vi "Emballage_BDD_Certificat_S1220009.vi"(0 "CODE BARRE":string, 11 "error in (no error)":errorcluster) -> (4 "Saved Report Path":path=path "C:/Users/ltinguely/Desktop/test model certificat calibration CHIPREG/CHIPREG_Certif_cali__2019-02-14_083035.doc", 15 "error out":errorcluster)   [LabVIEW 2020]
uses:
  Modules/FS/60_FS_Controles/60_FS_SetGet.ctl
  <vilib>/Utility/NIReport.llb/Report Type.ctl
  <vilib>/Utility/NIReport.llb/NI_report.lvclass
  <vilib>/Utility/NIReport.llb/NI_ReportGenerationCore.lvlib
  <vilib>/Utility/NIReport.llb/Word/NI_Word.lvclass
panel:
  out "Temps [s] 2":dbl
  out "Temps [s]":dbl
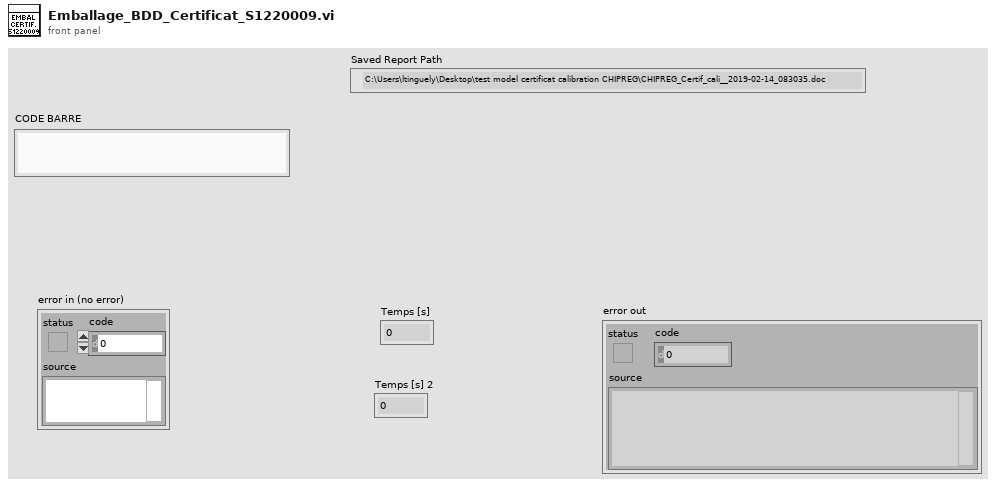
[diagram p1: front panel]
types:
  T1 = typedef "60_FS_SetGet.ctl" = enum16{"set", "get"}
  T2 = enum16{"maximized", "minimized", "normal", "no change"}
  T3 = typedef "NI_ReportGenerationCore.lvlib/Report Type.ctl" = enum16{"HTML", "Word", "Excel"}
  T4 = typedef "60_FS_CLT_Chemins.ctl" = cluster{"Racine_local":path, "Racine_reseau":path, "Racine_Support_Application":path, "Fichier_Journalisation":path, "Connexion_BDD_VSX":path, "Connexion_BDD_PLZ":path}
  T5 = typedef "Emballage_BDD_param_Produit.ctl" = cluster{"No_Valve_FAS":string, "suffixe":string, "designation":string, "indice_produit":string, "code_barre_fixe":string, "affiche_code_barre_client":string, "affiche_no_client":string, "Nb_vlve_par_carton":u16, "melange_des_lots_possible":string, "id_article":string, "Indice_Rev":string, "Famille":string, "date":string, "code_barre_fixe_Fin":string, "Longeur_No_Serie":string}
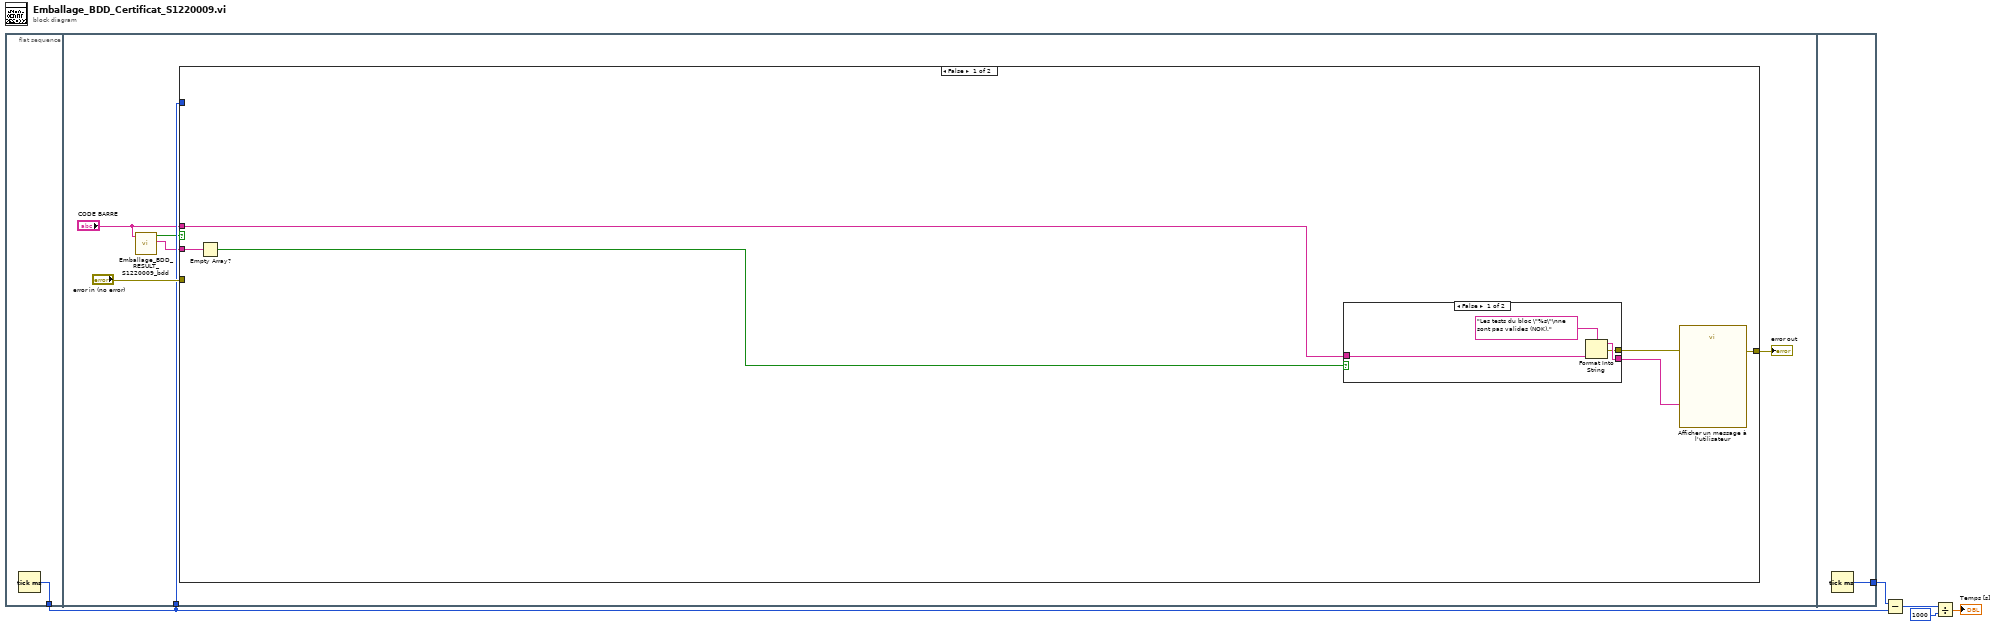
[diagram p0: block diagram]
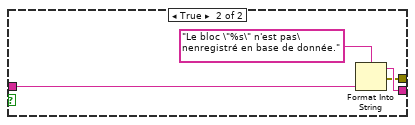
[diagram p2: hidden frame]
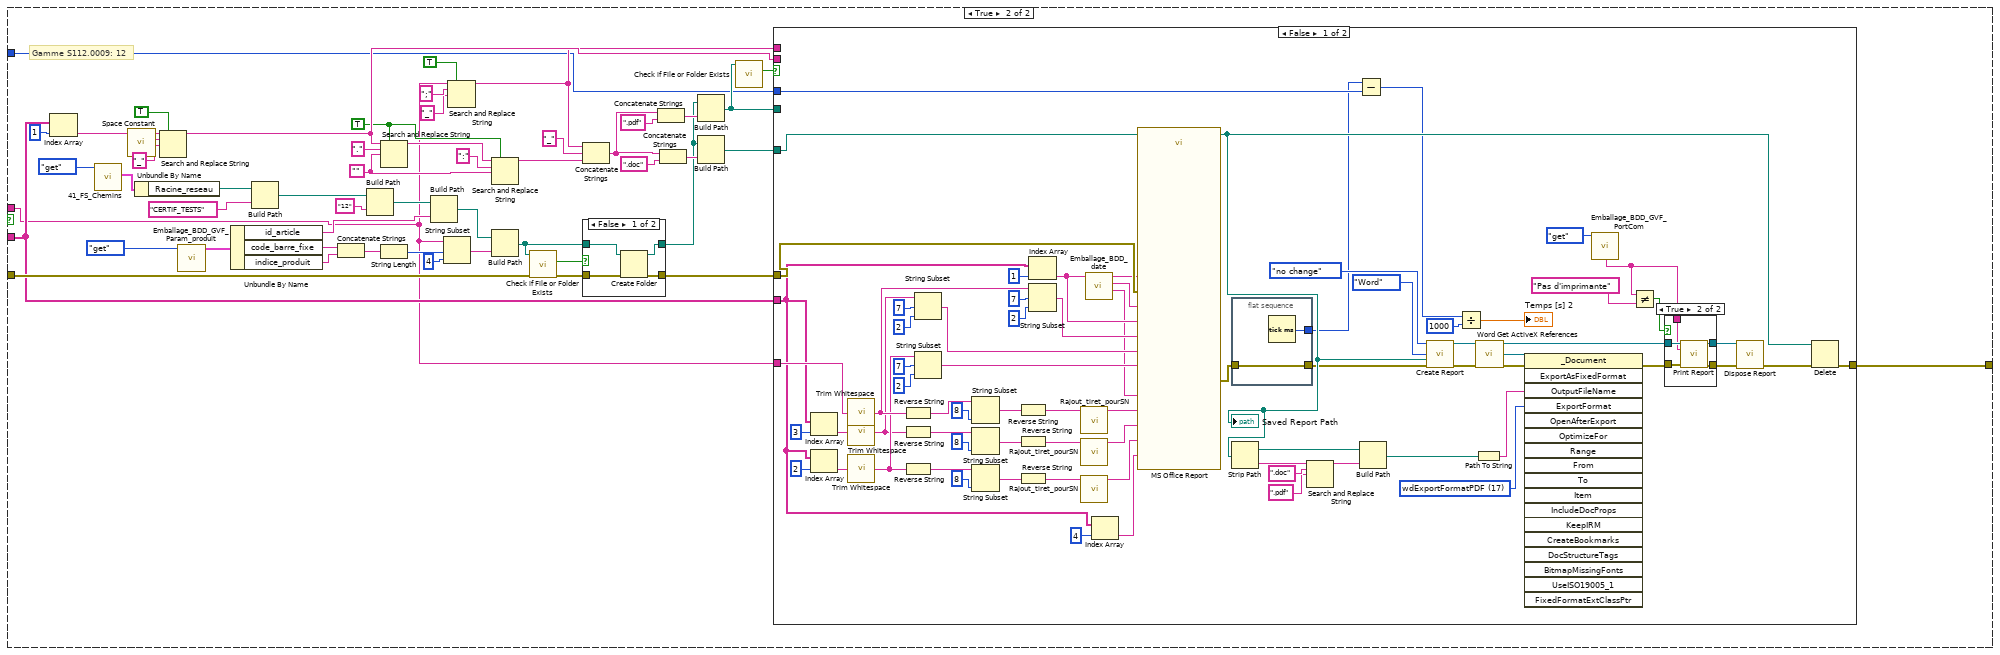
[diagram p3: hidden frame]
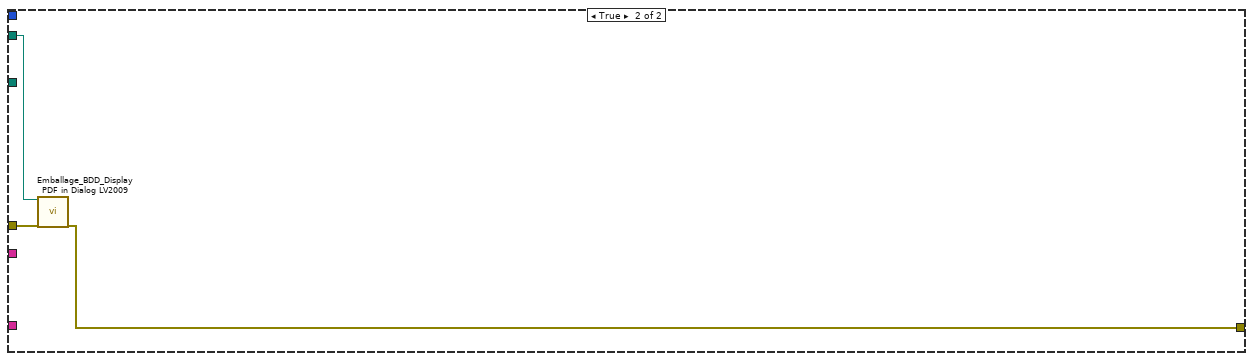
[diagram p6: hidden frame]
diagram:
  n1 = flat-sequence {
    tunnel: [w6] -> w1
    tunnel: w1 -> [w10]
    tunnel: [w171] -> w5
    frame #0 {
      n2 = Tick Count (ms)() -> (millisecond timer value=w6:u32)
    }
    frame #1 {
      n3 = call "Emballage_BDD_RESULT_S1220009_bdd.vi"("SN_PRODUIT"="CODE BARRE") -> ("dernière_donnée"=w7:string[], "result"=w8:bool)  [unwired: 8 in, 1 out]
      n4 = case shown="False" w8 {
        tunnel: [w18 w78] -> w12
        tunnel: "error in (no error)" -> [_ w44]
        tunnel: "CODE BARRE" -> [w15 w27]
        tunnel: w10 -> [_ w38]
        tunnel: w7 -> [w16 w35]
        frame False {
          n5 = Empty Array?(array=w16) -> (empty?=w17:bool)
          n6 = case shown="False" w17 {
            tunnel: w15 -> [w21 w24]
            tunnel: [w20 w25] -> w14
            tunnel: [w19 w23] -> w13
            frame False {
              n7 = Format Into String(format string="Les tests du bloc \"%s\"\nne sont pas valides (NOK)." ("chaîne de format"), w21) -> (resulting string=w20:string, error out=w19:errorcluster)  [unwired: 2 in]
            }
            frame True {
              n8 = Format Into String(format string="Le bloc \"%s\" n'est pas\nenregistré en base de donnée." ("chaîne de format"), w24) -> (resulting string=w25:string, error out=w23:errorcluster)  [unwired: 2 in]
            }
          }
          n9 = call "Afficher un message à l'utilisateur"("error in (no error)"=w13, "Message"=w14) -> ("error out"=w18:errorcluster)  [unwired: 8 in, 1 out]
        }
        frame True {
          w67 = TRUE ("tout remplacer ? (F)")
          w72 = ""
          # "Gamme S112.0009: 12"
          n10 = Index Array(array=w35, index=1 ("indice")) -> (element=w37:string)
          n11 = call "41_FS_Chemins.vi"("SetGet"=60_FS_SetGet."get") -> ("CLT_Chemins_out"=w53:T4)  [unwired: 9 in, 1 out]
          n12 = call <vilib>:"Space Constant.vi"() -> ("String"=w71:string)
          n13 = Unbundle By Name(w53) -> ("Racine_reseau"=w41:path)
          n14 = Search and Replace String(replace all?=TRUE ("tout remplacer ? (F)"), input string=w37, search string=w71, replace string="_" ("chaîne de remplacement (\"\")")) -> (result string=w68:string)  [unwired: 4 in, 3 out]
          n15 = call "Emballage_BDD_GVF_Param_produit.vi"("Énum"=enum16{"set", "get"}."get") -> ("CLS_param_produit"=w33:T5)  [unwired: 7 in, 3 out]
          n16 = Unbundle By Name(w33) -> ("id_article"=w32:string, "code_barre_fixe"=w31:string, "indice_produit"=w30:string)
          n17 = Build Path(base path=w41, name or relative path="CERTIF_TESTS" ("nom ou chemin relatif")) -> (appended path=w39:path)
          n18 = Concatenate Strings(w31, w30) -> (w29:string)
          n19 = Build Path(base path=w39, name or relative path="12" ("nom ou chemin relatif")) -> (appended path=w51:path)
          n20 = Search and Replace String(replace all?=w67, input string=w68, search string="." ("chaîne recherchée"), replace string=w72) -> (result string=w74:string)  [unwired: 4 in, 3 out]
          n21 = String Length(string=w29) -> (length=w28:i32)
          n22 = Build Path(base path=w51, name or relative path=w32) -> (appended path=w50:path)
          n23 = String Subset(string=w27, offset (0)=w28, length (rest)=4 ("longueur (reste)")) -> (substring=w49:string)
          n24 = Search and Replace String(replace all?=TRUE ("tout remplacer ? (F)"), input string=w27, search string=";" ("chaîne recherchée"), replace string="_" ("chaîne de remplacement (\"\")")) -> (result string=w56:string)  [unwired: 4 in, 3 out]
          n25 = Search and Replace String(replace all?=w67, input string=w74, search string=":" ("chaîne recherchée"), replace string=w72) -> (result string=w69:string)  [unwired: 4 in, 3 out]
          n26 = Build Path(base path=w50, name or relative path=w49) -> (appended path=w46:path)
          n27 = call <vilib>:"Check if File or Folder Exists.vi"("error in (no error)"=w44, "path"=w46) -> ("error out"=w45:errorcluster, "file or folder exists?"=w47:bool)  [unwired: 7 in, 1 out]
          n28 = Concatenate Strings(w56, "_", w69) -> (w63:string)
          n29 = case shown="False" w47 {
            tunnel: w46 -> [w82 w84]
            tunnel: w45 -> [w81 w83]
            tunnel: [w80 w83] -> w43
            tunnel: [w79 w84] -> w42
            frame False {
              n30 = Create Folder(path (use dialog)=w82, error in=w81) -> (created path=w79:path, error out=w80:errorcluster)  [unwired: 1 in, 1 out]
            }
            frame True {
            }
          }
          n31 = Concatenate Strings(w63, ".pdf" ("chaîne")) -> (w62:string)
          n32 = Concatenate Strings(w63, ".doc" ("chaîne")) -> (w64:string)
          n33 = Build Path(base path=w42, name or relative path=w62) -> (appended path=w59:path)
          n34 = Build Path(base path=w42, name or relative path=w64) -> (appended path=w77:path)
          n35 = call <vilib>:"Check if File or Folder Exists.vi"("path"=w59) -> ("file or folder exists?"=w60:bool)  [unwired: 8 in, 2 out]
          n36 = case shown="False" w60 {
            tunnel: [w156 w168] -> w78
            tunnel: w77 -> [w157 _]
            tunnel: w56 -> [_ _]
            tunnel: w68 -> [_ _]
            tunnel: w59 -> [_ w169]
            tunnel: w43 -> [w158 w170]
            tunnel: w38 -> [w134 _]
            tunnel: w35 -> [w86 _]
            tunnel: w27 -> [w109 _]
            frame False {
              w143 = 17 items=["wdExportFormatPDF"=17, "wdExportFormatXPS"=18] ("ExportFormat")
              n37 = Index Array(array=w86, index=3 ("indice")) -> (element=w122:string)
              n38 = Index Array(array=w86, index=2 ("indice")) -> (element=w123:string)
              n39 = call <vilib>:"Trim Whitespace.vi"("string"=w109) -> ("trimmed string"=w112:string)  [unwired: 1 in]
              n40 = call <vilib>:"Trim Whitespace.vi"("string"=w122) -> ("trimmed string"=w110:string)  [unwired: 1 in]
              n41 = call <vilib>:"Trim Whitespace.vi"("string"=w123) -> ("trimmed string"=w111:string)  [unwired: 1 in]
              n42 = Reverse String(1:w112) -> (0:w121:string)
              n43 = Reverse String(1:w110) -> (0:w115:string)
              n44 = Reverse String(1:w111) -> (0:w117:string)
              n45 = String Subset(string=w110, offset (0)=7, length (rest)=2 ("longueur (reste)")) -> (substring=w96:string)
              n46 = String Subset(string=w111, offset (0)=7, length (rest)=2 ("longueur (reste)")) -> (substring=w95:string)
              n47 = String Subset(string=w121, length (rest)=8 ("longueur (reste)")) -> (substring=w119:string)  [unwired: 1 in]
              n48 = String Subset(string=w115, length (rest)=8 ("longueur (reste)")) -> (substring=w113:string)  [unwired: 1 in]
              n49 = String Subset(string=w117, length (rest)=8 ("longueur (reste)")) -> (substring=w114:string)  [unwired: 1 in]
              n50 = Reverse String(1:w119) -> (0:w108:string)
              n51 = Reverse String(1:w113) -> (0:w106:string)
              n52 = Reverse String(1:w114) -> (0:w107:string)
              n53 = Index Array(array=w86, index=1 ("indice")) -> (element=w91:string)
              n54 = String Subset(string=w112, offset (0)=7, length (rest)=2 ("longueur (reste)")) -> (substring=w97:string)
              n55 = call "Rajout_tiret_pourSN.vi"("SN_Entrant"=w108) -> ("SN: avec -"=w94:string)  [unwired: 10 in]
              n56 = call "Rajout_tiret_pourSN.vi"("SN_Entrant"=w106) -> ("SN: avec -"=w93:string)  [unwired: 10 in]
              n57 = call "Rajout_tiret_pourSN.vi"("SN_Entrant"=w107) -> ("SN: avec -"=w92:string)  [unwired: 10 in]
              n58 = call "Emballage_BDD_date.vi"("Date"=w91) -> ("Date_jour"=w88:string, "Date_mois"=w89:string, "Date_annee"=w90:string)  [unwired: 8 in]
              n59 = Index Array(array=w86, index=4 ("indice")) -> (element=w85:string)
              n60 = call "MS Office Report"("Path to Save Report"=w157, "date_Annee"=w90, "date_Jour"=w88, "date_Mois"=w89, "Date_Test"=w91, "Index_bloc"=w97, "error in (no error)"=w158, "Index_Revolver_O2"=w96, "Index_Revolver_TG"=w95, "N_Série_Bloc"=w94, "N_Série_Revolver_O2"=w93, "N_Série_Revolver_TG"=w92, "Signature"=w85) -> ("Saved Report Path"=w140:path, "error out"=w138:errorcluster)  [unwired: 13 in]
              "Saved Report Path" <- w140
              n61 = flat-sequence {
                tunnel: [w167] -> w139
                tunnel: w138 -> [w167]
                tunnel: [w166] -> w133
                frame #0 {
                  n62 = Tick Count (ms)() -> (millisecond timer value=w166:u32)
                }
              }
              n63 = Strip Path(path=w140) -> (stripped path=w150:path, name=w147:string)
              n64 = Search and Replace String(input string=w147, search string=".doc" ("chaîne recherchée"), replace string=".pdf" ("chaîne de remplacement (\"\")")) -> (result string=w146:string)  [unwired: 5 in, 3 out]
              n65 = Subtract(x=w133, y=w134) -> (x-y=w137:u32)
              n66 = Build Path(base path=w150, name or relative path=w146) -> (appended path=w149:path)
              n67 = call <vilib>:"Create Report.vi"("window state (normal)"=T2."no change", "report type"=Report_Type."Word", "template (empty)"=w140, "error in (no error)"=w139) -> ("report out"=w153:refnum<class "NI_report.lvclass">, "error out"=w152:errorcluster)  [unwired: 10 in]
              n68 = Divide(x=w137, y=u32 1000) -> (x/y=→"Temps [s] 2":dbl)
              n69 = Path To String(path=w149) -> (string=w148:string)
              n70 = call <vilib>:"Word Get ActiveX References.vi"("report in"=w153, "error in (no error)"=w152) -> ("report out"=w101:refnum<class "NI_report.lvclass">, "Word._Document"=w151:refnum<k7>, "error out"=w142:errorcluster)  [unwired: 7 in, 4 out]
              n71 = invoke class="_Document" method="ExportAsFixedFormat"(reference=w151, error in=w142, "OutputFileName"=w148, "ExportFormat"=w143) -> (error out=w100:errorcluster)  [unwired: 14 in, 17 out]
              n72 = call "Emballage_BDD_GVF_PortCom.vi"("Énum"=enum16{"get", "set"}."get") -> ("Imprimante Certif."=w104:string)  [unwired: 8 in, 6 out]
              n73 = Not Equal?(x=w104, y="Pas d'imprimante") -> (x != y?=w103:bool)
              n74 = case shown="True" w103 {
                tunnel: [w159 w165] -> w99
                tunnel: w101 -> [w160 w164]
                tunnel: [w160 w163] -> w98
                tunnel: w100 -> [w159 w162]
                tunnel: w104 -> [_ w161]
                frame False {
                }
                frame True {
                  n75 = call-dynamic "Print Report.vi"("report in"=w164, "printer name (default)"=w161, "error in (no error)"=w162) -> ("report out"=w163:refnum<class "NI_report.lvclass">, "error out"=w165:errorcluster)  [unwired: 11 in]
                }
              }
              n76 = call-dynamic "Dispose Report.vi"("report in"=w98, "error in (no error)"=w99) -> ("error out"=w141:errorcluster)  [unwired: 13 in]
              n77 = Delete(path (use dialog)=w140, error in=w141) -> (error out=w156:errorcluster)  [unwired: 3 in, 2 out]
            }
            frame True {
              n78 = call "Emballage_BDD_Display PDF in Dialog LV2009.vi"("PDF file"=w169, "error in (no error)"=w170) -> ("error out"=w168:errorcluster)  [unwired: 17 in]
            }
          }
        }
      }
      "error out" <- w12
    }
    frame #2 {
      n79 = Tick Count (ms)() -> (millisecond timer value=w171:u32)
    }
  }
  n80 = Subtract(x=w5, y=w1) -> (x-y=w4:u32)
  n81 = Divide(x=w4, y=u32 1000) -> (x/y=→"Temps [s]":dbl)
